vi "Pack for gRPC.vi"(8 "error in":errorcluster, 9 "configuration / results":enum16{"Configuration", "Results"}(ring), 10 "data value":variant, 11 "measurement customizations in":refnum<class "Measurement Plugin.lvclass">) -> (0 "error out":errorcluster, 2 "any":T1, 3 "measurement customizations out":refnum<class "Measurement Plugin.lvclass">)   [LabVIEW 2024, in "Frequency Response (Discrete Sweep).lvlib" / "Measurement Plugin.lvclass"]
uses:
  Measurement Plugin.lvclass
  <vilib>/gRPC/LabVIEW gRPC Library/Shared/Any.ctl
  C:/Program Files/National Instruments/LabVIEW 2024/vi.lib/Plug-In SDKs/Measurements/Measurement Plugin Service/Measurement Plugin Service.lvclass
  Measurement Configuration.ctl
  Measurement Results.ctl
  <vilib>/gRPC/Generated APIs/ni/protobuf/types/RPC Messages/ni_protobuf_types_DoubleXYData.ctl
  2eca732d-dbaa-43bf-a7dd-ede2da65bc1b.vi
  a6012965-5700-4384-8228-972e71b6560c.vi
  <vilib>/gRPC/LabVIEW gRPC Library/Server API/Translate Protobuf Error.vi
  <vilib>/AdvancedString/1D String Array to Delimited String.vi
  <vilib>/gRPC/LabVIEW gRPC Library/Server API/Server/Get Server DLL Path.vi
  Frequency Response (Discrete Sweep).lvlib
  <vilib>/gRPC/Generated APIs/ni/protobuf/types/ni.protobuf.types.lvlib
  <vilib>/Plug-In SDKs/Measurements/Measurement Plugin Service/Measurement Plugin Service.lvclass
  <vilib>/gRPC/LabVIEW gRPC Library/grpc-lvsupport-release.lvlib
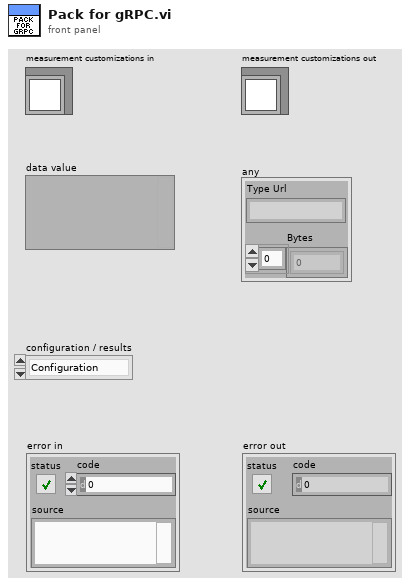
[diagram p1: front panel]
types:
  T1 = typedef "grpc-lvsupport-release.lvlib/Any.ctl" = cluster{"Type Url":string, "Bytes":u8[]}
  T2 = typedef "grpc-lvsupport-release.lvlib/grpcId.ctl" = u64
  T3 = typedef "Frequency Response (Discrete Sweep).lvlib/Measurement Configuration.ctl" = cluster{"sample rate":dbl, "ao stimulus channel":string, "ao range":dbl, "ao terminal configuration":i32, "ai reference channel":string, "ai ref range":dbl, "ai reference terminal configuration":i32, "ai response channel":string, "ai response range":dbl, "ai response terminal configuration":i32, "amplitude":dbl, "start frequency":dbl, "stop frequency":dbl, "number of steps":i32, "profile":enum32{"Linear", "Logarithmic"}, "measurement time":dbl, "measurement cycles":i32}
  T4 = typedef "Frequency Response (Discrete Sweep).lvlib/Measurement Results.ctl" = cluster{"current frequency":dbl, "waveforms file path":string, "reference RMS level":T5, "response RMS level":T5, "FRF magnitude":T5, "FRF phase":T5, "THD":T5, "h2":T5, "h3":T5, "h4":T5, "h5":T5, "THDN":T5}
  T5 = typedef "ni.protobuf.types.lvlib/ni_protobuf_types_DoubleXYData.ctl" = cluster{"x_data":dbl[], "y_data":dbl[]}
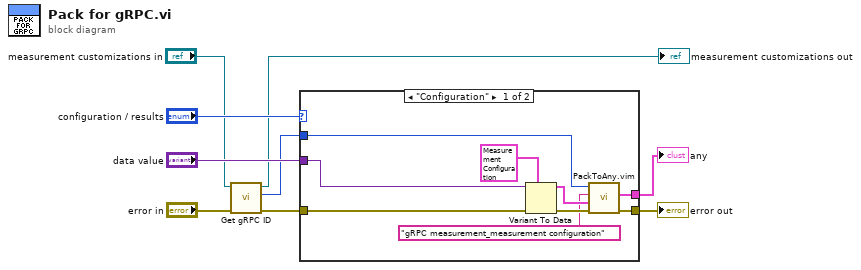
[diagram p0: block diagram]
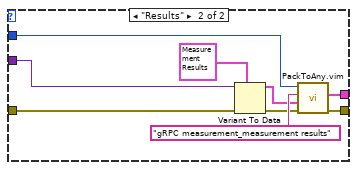
[diagram p2: hidden frame]
diagram:
  n1 = call <vilib>:"Get gRPC ID.vi"("error in"="error in", "measurement plugin service in"="measurement customizations in") -> ("error out"=w4:errorcluster, "gRPC ID"=w1:T2, "measurement plugin service out"=→"measurement customizations out":refnum<class "Measurement Plugin.lvclass">)  [unwired: 7 in]
  n2 = case shown="\"Configuration\"" "configuration / results" {
    tunnel: w4 -> [w18 w27]
    tunnel: "data value" -> [w17 w26]
    tunnel: w1 -> [w14 w22]
    tunnel: [w16 w24] -> w8
    tunnel: [w15 w23] -> w7
    frame "Configuration" {
      n3 = Variant To Data(error in=w18, type=T3 {"sample rate"=1.2, "ao stimulus channel"="Lorem ipsum dolor sit", "ao range"=32.0, "ao terminal configuration"=32, "ai reference channel"="Dev1/ai0", "ai ref range"=64.0, "ai reference terminal configuration"=-32, "ai response channel"="Dev1/ai1", "ai response range"=-64.0, "ai response terminal configuration"=-64, "amplitude"=1.0, "start frequency"=1.0, "stop frequency"=1.0, "number of steps"=1, "profile"=enum."Logarithmic", "measurement time"=0.001, "measurement cycles"=10} ("measurement configuration"), Variant=w17) -> (data=w13:T3, error out=w12:errorcluster)
      n4 = call "PackToAny.vim"("error in"=w12, "Data To Pack"=w13, "Message Type"="gRPC measurement_measurement configuration", "gRPCid in"=w14) -> ("error out"=w16:errorcluster, "Any"=w15:T1)  [unwired: 5 in, 1 out]
    }
    frame "Results" {
      n5 = Variant To Data(error in=w27, type=T4 {"current frequency"=0.0, "waveforms file path"="Empty", "reference RMS level"={"x_data"=[], "y_data"=[]}, "response RMS level"={"x_data"=[], "y_data"=[0.0]}, "FRF magnitude"={"x_data"=[0.0], "y_data"=[0.0]}, "FRF phase"={"x_data"=[0.0], "y_data"=[]}, "THD"={"x_data"=[], "y_data"=[]}, "h2"={"x_data"=[], "y_data"=[]}, "h3"={"x_data"=[], "y_data"=[]}, "h4"={"x_data"=[], "y_data"=[]}, "h5"={"x_data"=[], "y_data"=[]}, "THDN"={"x_data"=[], "y_data"=[]}} ("Measurement Results"), Variant=w26) -> (data=w20:T4, error out=w19:errorcluster)
      n6 = call "PackToAny.vim"("error in"=w19, "Data To Pack"=w20, "Message Type"="gRPC measurement_measurement results", "gRPCid in"=w22) -> ("error out"=w24:errorcluster, "Any"=w23:T1)  [unwired: 5 in, 1 out]
    }
  }
  "error out" <- w8
  "any" <- w7
